vi "Display Elements RT Test Panel.vi"() -> ()   [LabVIEW 2019]
uses:
  Graph/Public/Controls/Fill To.ctl
  Graph/Public/Controls/Range.ctl
  Display Utilities/Public/Controls/2D Dimensions.ctl
  Display/Public/Controls/RGB Gains.ctl
  Display Utilities/Public/Controls/2D Coordinates.ctl
  Pixel/Pixel.lvclass
  C:/Users/goo13/Documents/GIT Local/myRIO-Neopixel/Source/RT/Display Element/Display Element.lvclass
  Square/Square.lvclass
  String/String.lvclass
  Graph/Graph.lvclass
  <vilib>/FPGAPlugInAG/myRIO-1900/niLvFpga_Open_myRIO-1900.vi
  <vilib>/rvi/interface/common/dynamic/niFpgaDynamicAddResources.vi
  <vilib>/Utility/error.llb/Error Cluster From Error Code.vi
  <vilib>/rvi/errors/niLvFpgaAdjustHostInterfaceError.vi
  <vilib>/FPGAPlugInAG/Dynamic/niLvFpga_Close_Dynamic.vi
  <vilib>/rvi/interface/nirviOpenFPGA/nirviOpenFPGA.xnode
  FPGA Bitfiles/myrio-neopixel_FPGATarget_TestNeopixel_-8uHP6HNTAw.lvbitx
  <vilib>/rvi/interface/nirviReadWriteControl/nirviReadWriteControl.xnode
  <vilib>/rvi/interface/nirviMethod/nirviMethod.xnode
  <vilib>/rvi/interface/nirviCloseFPGA/nirviCloseFPGA.xnode
  Display Element/Display Element.lvclass
  Display/Display.lvclass
  Display Utilities/Display Utilities.lvlib
  <vilib>/FPGAPlugInAG/Dynamic/niLvFpga_WriteFifo_Dynamic.vi
  <vilib>/rvi/errors/niLvFpgaMergeErrorWithErrorCode.vi
  NiFpgaLv.dll
  <vilib>/rvi/interface/Simulation/niFpgaSimulationCallBeginRW.vi
panel:
  in  "Intensity":sgl(slide)=0.5 scale=0.0..1.0
  out "Error Out":errorcluster
  in  "FPS":u32(slide)=40 scale=0.0..100.0
  in  "Display X":i32=24 caption="X"
  in  "Display Y":i32=8 caption="Y"
  in  "Position X":i32 caption="X"
  in  "Position Y":i32 caption="Y"
  in  "Force X":i32 caption="X"
  in  "Force Y":i32 caption="Y"
  in  "Tag":string
  in  "Layer":u32
  in  "Delete If Outside Bounds":bool=TRUE
  in  "Color":u32(colorbox)
  in  "Create Button":bool
  in  "Element Type":enum32{"Pixel", "Square", "String", "Graph"}(tab)
  in  "Trace":i32
  in  "Height":u32
  in  "Width":u32
  in  "Text":string
  in  "Width G":u32 caption="Width"
  in  "Height G":u32 caption="Height"
  in  "Data":i32[](array[numeric])
  in  "Fill To":T1
  in  "Range":T2
  out "Frame":u32[][](array[colorbox])
  in  "stop":bool
  # "Display Settings"
  # "Display Size"
  # "Display Elements Creation"
  # "Position"
  # "Force"
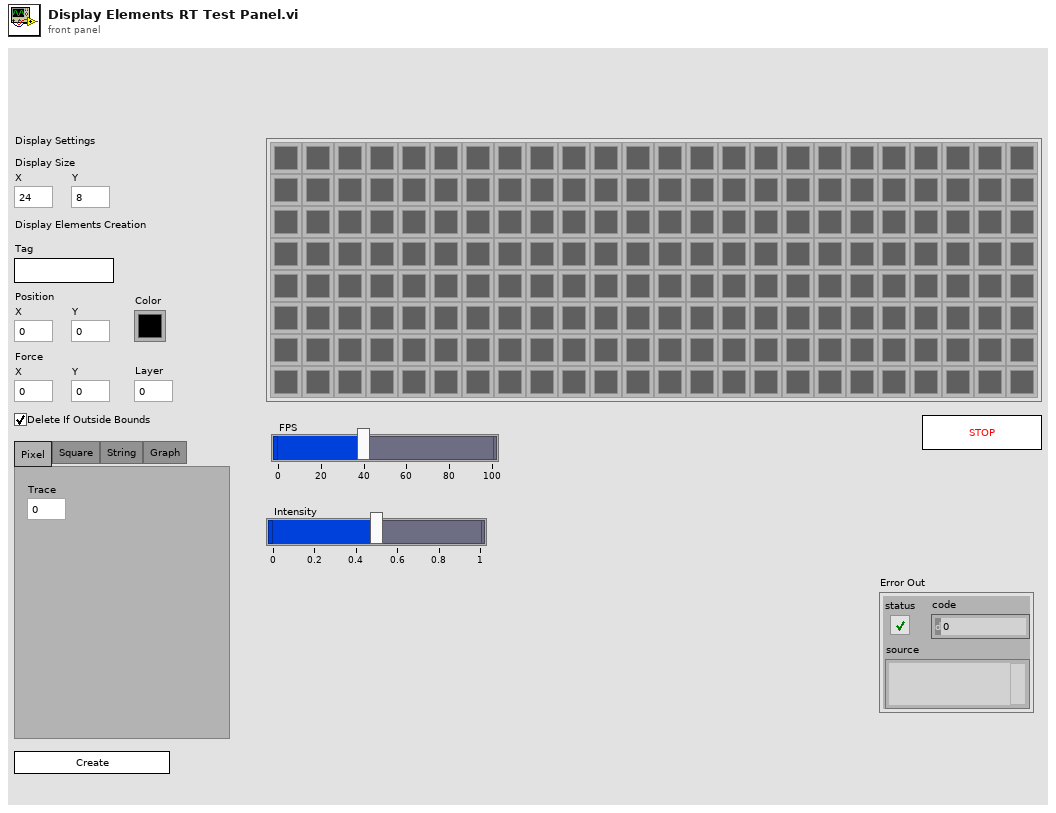
[diagram p1: front panel]
types:
  T1 = typedef "Graph.lvclass/Fill To.ctl" = enum16{"None", "Inf", "-Inf"}
  T2 = typedef "Graph.lvclass/Range.ctl" = cluster{"Maximum":dbl, "Minimum":dbl}
  T3 = typedef "Display Utilities.lvlib/2D Dimensions.ctl" = cluster{"Width":i32, "Height":i32}
  T4 = typedef "Display.lvclass/RGB Gains.ctl" = cluster{"Red":sgl, "Green":sgl, "Blue":sgl}
  T5 = typedef "Display Utilities.lvlib/2D Coordinates.ctl" = cluster{"X":i32, "Y":i32}
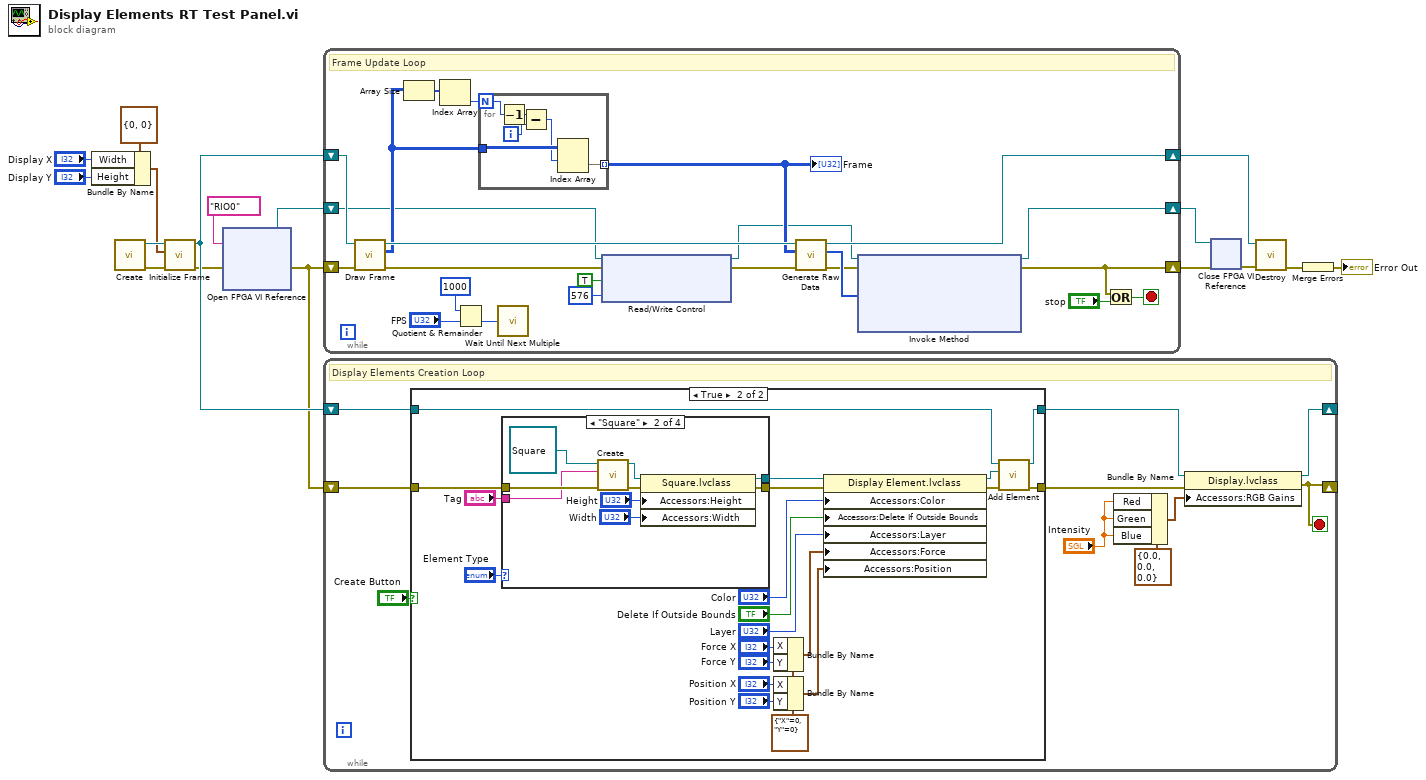
[diagram p0: block diagram]
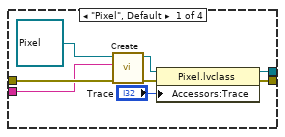
[diagram p3: hidden frame]
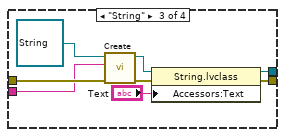
[diagram p4: hidden frame]
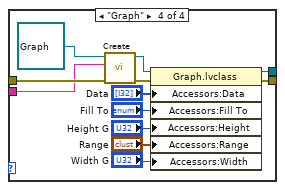
[diagram p5: hidden frame]
diagram:
  n1 = Bundle By Name(cluster=T3 {"Width"=0, "Height"=0} ("Size"), "Width"="Display X", "Height"="Display Y") -> (w10:T3)
  n2 = call "Create.vi"() -> ("Error Out"=w15:errorcluster, "Screen Out"=w16:refnum<class "Display.lvclass">)  [unwired: 10 in]
  n3 = call "Initialize Frame.vi"("Error In"=w15, "Size"=w10, "Display In"=w16) -> ("Error Out"=w8:errorcluster, "Display Out"=w14:refnum<class "Display.lvclass">)  [unwired: 7 in]
  n4 = xnode "Open FPGA VI Reference"("error in"=w8, "resource name"=tag "RIO0") -> ("FPGA VI Reference Out"=w6:refnum<k20>, "error out"=w7:errorcluster)
  n5 = while {
    shift-right: [w22] -> w5
    shift-left: w7 -> [w36]
    shift-right: [w27] -> w17
    shift-left: w14 -> [w35]
    shift-right: [w23] -> w4
    shift-left: w6 -> [w21]
    stop <- w39 stop-if-true
    # "Frame Update Loop"
    n6 = call "Draw Frame.vi"("Error In"=w36, "Display In"=w35) -> ("Error Out"=w20:errorcluster, "Frame"=w26:u32[][], "Display Out"=w30:refnum<class "Display.lvclass">)  [unwired: 7 in]
    n7 = Array Size(array=w26) -> (size(s)=w38:i32[])
    n8 = Index Array(array=w38) -> (element=w37:i32)  [unwired: 1 in]
    n9 = Quotient & Remainder(x=u32 1000 ("y"), y="FPS") -> (floor(x/y)=w34:u32)  [unwired: 1 out]
    n10 = for {
      N: w37 -> [w43]
      tunnel: w26 -> [w45]
      tunnel: [w41] -> w25 mode=indexing
      i -> [w46]
      n11 = Decrement(x=w43) -> (x-1=w42:i32)
      n12 = Subtract(x=w42, y=w46) -> (x-y=w44:i32)
      n13 = Index Array(array=w45, index (row)=w44) -> (element=w41:u32[])  [unwired: 1 in]
    }
    "Frame" <- w25
    n14 = call "Wait Until Next Multiple"("Count(mSec)"=w34) -> ()  [unwired: 1 out]
    n15 = xnode "Read/Write Control"("FPGA VI Reference In"=w21, "error in"=w20, "Update"=TRUE, "Number Of Elements"=576) -> ("FPGA VI Reference Out"=w18:refnum<k20>, "error out"=w19:errorcluster)
    n16 = call "Generate Raw Data.vi"("Error In"=w19, "Matrix"=w25, "Display In"=w30) -> ("Error Out"=w24:errorcluster, "Raw Data"=w31:u8[], "Display Out"=w27:refnum<class "Display.lvclass">)  [unwired: 6 in]
    n17 = xnode "Invoke Method"("FPGA VI Reference In"=w18, "error in"=w24, "Data"=w31) -> ("FPGA VI Reference Out"=w23:refnum<k20>, "error out"=w22:errorcluster)  [unwired: 1 in, 1 out]
    n18 = Or(x=w22, y="stop") -> (x .or. y?=w39:bool)
  }
  n19 = while {
    shift-right: [w48] -> _
    shift-left: w14 -> [w56]
    shift-right: [w47] -> _
    shift-left: w7 -> [w55]
    stop <- w47 stop-if-true
    # "Display Elements Creation Loop"
    n20 = case shown="True" "Create Button" {
      tunnel: w56 -> [w57 w78]
      tunnel: w55 -> [w58 w74]
      tunnel: [w57 w77] -> w49
      tunnel: [w58 w76] -> w50
      frame False {
      }
      frame True {
        w66 = T5 {"X"=0, "Y"=0} ("Force")
        n21 = case shown="\"Square\"" "Element Type" {
          tunnel: w74 -> [w85 w94 w103 w115]
          tunnel: [w80 w89 w97 w111] -> w73
          tunnel: [w81 w88 w98 w112] -> w72
          tunnel: "Tag" -> [w79 w87 w96 w110]
          frame "Pixel", Default {
            n22 = call-dynamic "Create.vi"("Error In"=w85, "Tag"=w79, "Pixel In"=refnum<class "Pixel.lvclass"> refnum ("Pixel.lvclass")) -> ("Error Out"=w83:errorcluster, "Pixel Out"=w84:refnum<class "Pixel.lvclass">)  [unwired: 7 in]
            n23 = property class="Pixel.lvclass"(reference=w84, error in=w83, "Accessors:Trace"="Trace") -> (reference out=w81:refnum<class "Pixel.lvclass">, error out=w80:errorcluster)
          }
          frame "Square" {
            n24 = call-dynamic "Create.vi"("Error In"=w94, "Tag"=w87, "Square In"=refnum<class "Square.lvclass"> refnum ("Square.lvclass")) -> ("Error Out"=w92:errorcluster, "Square Out"=w93:refnum<class "Square.lvclass">)  [unwired: 7 in]
            n25 = property class="Square.lvclass"(reference=w93, error in=w92, "Accessors:Height"="Height", "Accessors:Width"="Width") -> (reference out=w88:refnum<class "Square.lvclass">, error out=w89:errorcluster)
          }
          frame "String" {
            n26 = call-dynamic "Create.vi"("Error In"=w103, "Tag"=w96, "Pixel In"=refnum<class "String.lvclass"> refnum ("String.lvclass")) -> ("Error Out"=w100:errorcluster, "Pixel Out"=w101:refnum<class "String.lvclass">)  [unwired: 7 in]
            n27 = property class="String.lvclass"(reference=w101, error in=w100, "Accessors:Text"="Text") -> (reference out=w98:refnum<class "String.lvclass">, error out=w97:errorcluster)
          }
          frame "Graph" {
            n28 = call-dynamic "Create.vi"("Error In"=w115, "Tag"=w110, "Graph In"=refnum<class "Graph.lvclass"> refnum ("Graph.lvclass")) -> ("Error Out"=w113:errorcluster, "Graph Out"=w114:refnum<class "Graph.lvclass">)  [unwired: 7 in]
            n29 = property class="Graph.lvclass"(reference=w114, error in=w113, "Accessors:Data"="Data", "Accessors:Fill To"="Fill To", "Accessors:Height"="Height G", "Accessors:Range"="Range", "Accessors:Width"="Width G") -> (reference out=w112:refnum<class "Graph.lvclass">, error out=w111:errorcluster)
          }
        }
        n30 = Bundle By Name(cluster=w66, "X"="Force X", "Y"="Force Y") -> (w65:T5)
        n31 = Bundle By Name(cluster=w66, "X"="Position X", "Y"="Position Y") -> (w64:T5)
        n32 = property class="Display Element.lvclass"(reference=w72, error in=w73, "Accessors:Color"="Color", "Accessors:Delete If Outside Bounds"="Delete If Outside Bounds", "Accessors:Layer"="Layer", "Accessors:Force"=w65, "Accessors:Position"=w64) -> (reference out=w70:refnum<class "Display Element.lvclass">, error out=w69:errorcluster)
        n33 = call "Add Element.vi"("Error In"=w69, "New Element"=w70, "Display In"=w78) -> ("Error Out"=w76:errorcluster, "Display Out"=w77:refnum<class "Display.lvclass">)  [unwired: 7 in]
      }
    }
    n34 = Bundle By Name(cluster=T4 {"Red"=0.0, "Green"=0.0, "Blue"=0.0} ("RGB Gains"), "Red"="Intensity", "Green"="Intensity", "Blue"="Intensity") -> (w53:T4)
    n35 = property class="Display.lvclass"(reference=w49, error in=w50, "Accessors:RGB Gains"=w53) -> (reference out=w48:refnum<class "Display.lvclass">, error out=w47:errorcluster)
  }
  n36 = xnode "Close FPGA VI Reference"("FPGA VI Reference In"=w4, "error in"=w5) -> ("error out"=w3:errorcluster)
  n37 = call "Destroy.vi"("Error In"=w3, "Display In"=w17) -> ("Error Out"=w2:errorcluster)  [unwired: 9 in]
  n38 = Merge Errors(w2) -> (→"Error Out":errorcluster)
